vi "SwerveEncoderMain.vi"(3 "Control Mode":T1) -> (0 "swerveDistance":dbl, 1 "driveDistance":dbl)   [LabVIEW 2017]
uses:
  Control Mode.ctl
  <vilib>/Rock Robotics/SystemInterfaces/DIO/FPGA_DIOChannel.ctl
  <vilib>/Rock Robotics/WPI/Encoder/WPI_EncoderDevRef.ctl
  <vilib>/Rock Robotics/SystemInterfaces/Encoder/FPGA_EncoderIdx.ctl
  <vilib>/Rock Robotics/SystemInterfaces/Counter/FPGA_CounterCtrSystemIndex.ctl
  <vilib>/Rock Robotics/WPI/Encoder/WPI_EncoderType.ctl
  <vilib>/Rock Robotics/WPI/Counter/WPI_CounterDigitalInputToDigitalSource.vi
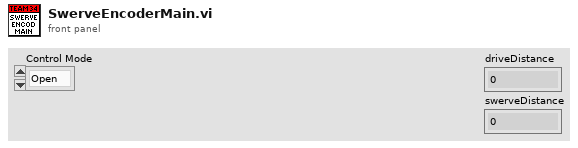
[diagram p1: front panel]
types:
  T1 = typedef "Control Mode.ctl" = enum16{"Open", "Control"}
  T2 = typedef "WPI_EncoderDevRef.ctl" = cluster{"DevStatus":errorcluster, "EncoderIndex":T3, "CounterIndex":T4, "DistancePerCount":dbl, "Decoding Type":T5}
  T3 = typedef "FPGA_EncoderIdx.ctl" = enum8{"Enc 0", "Enc 1", "Enc 2", "Enc 3", "Enc 4", "Enc 5", "Enc 6", "Enc 7", "Invalid"}
  T4 = typedef "FPGA_CounterCtrSystemIndex.ctl" = enum8{"Ctr 0", "Ctr 1", "Ctr 2", "Ctr 3", "Ctr 4", "Ctr 5", "Ctr 6", "Ctr 7", "Invalid"}
  T5 = typedef "WPI_EncoderType.ctl" = enum16{"1x", "2x", "4x"}
  T6 = cluster{"swerveEncoderDefRef":T2, "driveEncoderDefRef":T2}
  T7 = typedef "FPGA_DIOChannel.ctl" = enum8{"DIO 0", "DIO 1", "DIO 2", "DIO 3", "DIO 4", "DIO 5", "DIO 6", "DIO 7", "DIO 8", "DIO 9", "DIO MXP 0", "DIO MXP 1", "DIO MXP 2", "DIO MXP 3", "DIO MXP 4", "DIO MXP 5", "DIO MXP 6", "DIO MXP 7", "DIO MXP 8", "DIO MXP 9", "DIO MXP 10", "DIO MXP 11", "DIO MXP 12", "DIO MXP 13", "DIO MXP 14", "DIO MXP 15", "SPI Port CS1", "SPI Port CS2", "SPI Port CS3", "SPI Port MISO", "SPI Port MOSI", "Invalid"}
  T8 = typedef "WPI_DigitalInputDevRef.ctl" = cluster{"DevStatus":errorcluster, "DIO Channel":T7}
  T9 = typedef "FPGA_CounterEncoderSourceConvertionLVSourceType.ctl" = cluster{"DevStatus":errorcluster, "AnalogTriggerMode?":bool, "DigitalMode":cluster{"DIO Channel":T10}, "AnalogTriggerMode":cluster{"AnalogTriggerIndex":T11, "OutputType":T12}}
  T10 = typedef "FPGA_DIODigitalSourceChannel.ctl" = enum8{"DIO 0", "DIO 1", "DIO 2", "DIO 3", "DIO 4", "DIO 5", "DIO 6", "DIO 7", "DIO 8", "DIO 9", "DIO MXP 0", "DIO MXP 1", "DIO MXP 2", "DIO MXP 3", "DIO MXP 4", "DIO MXP 5", "DIO MXP 6", "DIO MXP 7", "DIO MXP 8", "DIO MXP 9", "DIO MXP 10", "DIO MXP 11", "DIO MXP 12", "DIO MXP 13", "DIO MXP 14", "DIO MXP 15", "Disabled"}
  T11 = typedef "FPGA_AnalogTriggerIndex.ctl" = enum8{"Trig 0", "Trig 1", "Trig 2", "Trig 3", "Trig 4", "Trig 5", "Trig 6", "Trig 7", "Invalid"}
  T12 = typedef "FPGA_AnalogTriggerOutType.ctl" = enum16{"InWindow", "TriggerState", "Rising", "Falling"}
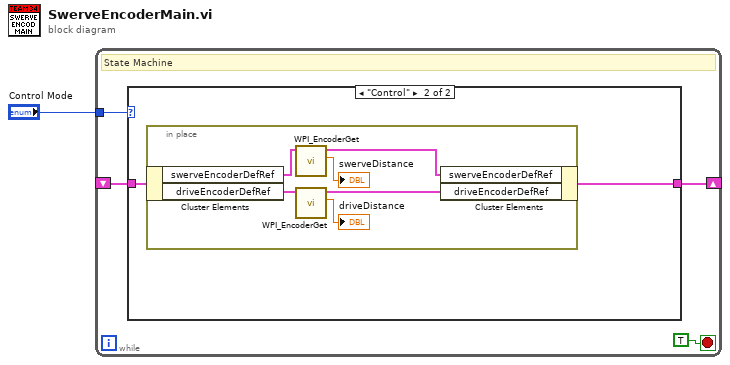
[diagram p0: block diagram]
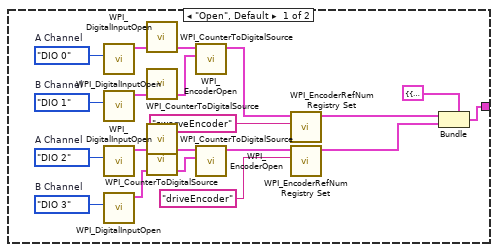
[diagram p2: hidden frame]
diagram:
  n1 = while {
    tunnel: "Control Mode" -> [w4]
    shift-right: [w3] -> _
    shift-left: _ -> [w2]
    stop <- TRUE stop-if-true
    # "State Machine"
    n2 = case shown="\"Control\"" w4 {
      tunnel: [w6 w26] -> w3
      tunnel: w2 -> [_ w27]
      frame "Open", Default {
        w19 = FPGA_DIOChannel."DIO 3"  # B Channel
        w18 = FPGA_DIOChannel."DIO 2"  # A Channel
        w25 = FPGA_DIOChannel."DIO 1"  # B Channel
        w24 = FPGA_DIOChannel."DIO 0"  # A Channel
        n3 = call <vilib>:"WPI_DigitalInputOpen.vi"("DIO Channel"=w24) -> ("DigitalInputDevRef"=w21:T8)  [unwired: 1 in, 9 out]
        n4 = call <vilib>:"WPI_DigitalInputOpen.vi"("DIO Channel"=w25) -> ("DigitalInputDevRef"=w22:T8)  [unwired: 1 in, 9 out]
        n5 = call <vilib>:"WPI_DigitalInputOpen.vi"("DIO Channel"=w18) -> ("DigitalInputDevRef"=w15:T8)  [unwired: 1 in, 9 out]
        n6 = call <vilib>:"WPI_DigitalInputOpen.vi"("DIO Channel"=w19) -> ("DigitalInputDevRef"=w16:T8)  [unwired: 1 in, 9 out]
        n7 = call-poly <vilib>:"WPI_CounterToDigitalSource.vi"("DigitalInputDevRef"=w21) -> ("Digital Source"=w20:T9)  [unwired: 6 out]
        n8 = call-poly <vilib>:"WPI_CounterToDigitalSource.vi"("DigitalInputDevRef"=w22) -> ("Digital Source"=w23:T9)  [unwired: 6 out]
        n9 = call-poly <vilib>:"WPI_CounterToDigitalSource.vi"("DigitalInputDevRef"=w15) -> ("Digital Source"=w14:T9)  [unwired: 6 out]
        n10 = call-poly <vilib>:"WPI_CounterToDigitalSource.vi"("DigitalInputDevRef"=w16) -> ("Digital Source"=w17:T9)  [unwired: 6 out]
        n11 = call <vilib>:"WPI_EncoderOpen.vi"("BSource"=w23, "ASource"=w20) -> ("EncoderDevRef"=w12:T2)  [unwired: 6 in, 3 out]
        n12 = call <vilib>:"WPI_EncoderOpen.vi"("BSource"=w17, "ASource"=w14) -> ("EncoderDevRef"=w13:T2)  [unwired: 6 in, 3 out]
        n13 = call <vilib>:"WPI_EncoderRefNum Registry Set.vi"("refnum name"="swerveEncoder", "EncoderDevRef"=w12) -> ("EncoderDevRef"=w9:T2)  [unwired: 8 in, 1 out]
        n14 = call <vilib>:"WPI_EncoderRefNum Registry Set.vi"("refnum name"="driveEncoder", "EncoderDevRef"=w13) -> ("EncoderDevRef"=w8:T2)  [unwired: 8 in, 1 out]
        n15 = Bundle(cluster=T6 {"swerveEncoderDefRef"={"DevStatus"={"status"=FALSE, "code"=0, "source"=""}, "EncoderIndex"=enum."Enc 0", "CounterIndex"=enum."Ctr 0", "DistancePerCount"=0.0, "Decoding Type"=enum."1x"}, "driveEncoderDefRef"={"DevStatus"={"status"=FALSE, "code"=0, "source"=""}, "EncoderIndex"=enum."Enc 0", "CounterIndex"=enum."Ctr 0", "DistancePerCount"=0.0, "Decoding Type"=enum."1x"}}, "swerveEncoderDefRef"=w9, "driveEncoderDefRef"=w8) -> (w6:T6)
      }
      frame "Control" {
        n16 = in-place {
          n17 = in-place-cluster #1(w27) -> ("swerveEncoderDefRef"=w33:T2, "driveEncoderDefRef"=w31:T2)
          n18 = call <vilib>:"WPI_EncoderGet.vi"("EncoderDevRef"=w33) -> ("Distance"=→"swerveDistance":dbl, "EncoderDevRef"=w32:T2)  [unwired: 5 in, 4 out]
          n19 = call <vilib>:"WPI_EncoderGet.vi"("EncoderDevRef"=w31) -> ("Distance"=→"driveDistance":dbl, "EncoderDevRef"=w30:T2)  [unwired: 5 in, 4 out]
          n20 = in-place-cluster #1("swerveEncoderDefRef"=w32, "driveEncoderDefRef"=w30) -> (w26:T6)
        }
      }
    }
  }
